vi "Path Manager.vi"   [LabVIEW 2026, in "PXI_Common.lvlib"]
uses:
  PXI_Common.lvlib
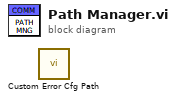
[diagram p0: block diagram]
diagram:
  n1 = call "Custom Error Cfg Path.vi"() -> ()  [unwired: 10 in, 2 out]
